vi "Example Input.vi"() -> ()   [LabVIEW 2010]
uses:
  C:/tf/play/labview/Tinkerforge.dll
  Tinkerforge.dll
panel:
  out "value mask":bool[](array[boolean])
  in  "uid":string="cnq"
  in  "port":i32=4223
  in  "host":string="localhost"
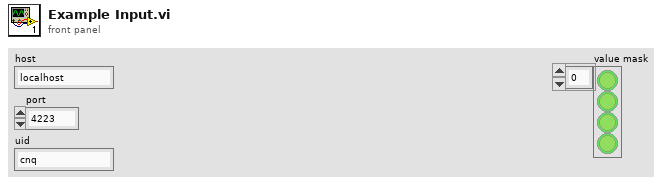
[diagram p1: front panel]
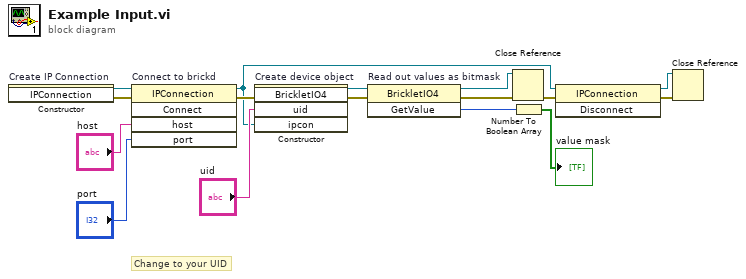
[diagram p0: block diagram]
diagram:
  # "Change to your UID"
  n1 = constructor on="Create IP Connection" class="IPConnection"() -> (reference out=w16:refnum<k24>, error out=w4:errorcluster)  [unwired: 3 in, 1 out]
  n2 = invoke on="Connect to brickd" class="IPConnection" method="Connect"(reference=w16, error in=w4, "host"="host", "port"="port") -> (reference out=w6:refnum<k24>, error out=w12:errorcluster)  [unwired: 1 in, 3 out]
  n3 = constructor on="Create device object" class="BrickletIO4"(error in=w12, "uid"="uid", "ipcon"=w6) -> (reference out=w11:refnum<k24>, error out=w1:errorcluster)  [unwired: 2 in, 3 out]
  n4 = invoke on="Read out values as bitmask" class="BrickletIO4" method="GetValue"(reference=w11, error in=w1) -> (reference out=w9:refnum<k24>, error out=w10:errorcluster, "GetValue"=w2:u8)  [unwired: 1 in]
  n5 = Close Reference(reference=w9, error in (no error)=w10) -> (error out=w8:errorcluster)
  n6 = Number To Boolean Array(number=w2) -> (Boolean array=→"value mask":bool[])
  n7 = invoke class="IPConnection" method="Disconnect"(reference=w6, error in=w8) -> (reference out=w5:refnum<k24>, error out=w7:errorcluster)  [unwired: 1 in, 1 out]
  n8 = Close Reference(reference=w5, error in (no error)=w7) -> ()  [unwired: 1 out]
